vi "Generate Field and Goal Posts.vi"(6 "Height":i16, 11 "Game Board in":refnum<class "Game Board.lvclass">) -> (2 "Goal post out":T1(array[cluster]), 3 "Field limit out":T1(array[cluster]))   [LabVIEW 2021, in "Game Board.lvclass"]
doc: "MIT Licence\nCopyright (c) 2024 David Grollier"
uses:
  Game Board.lvclass
  Game Board.lvclass/Game Board.ctl
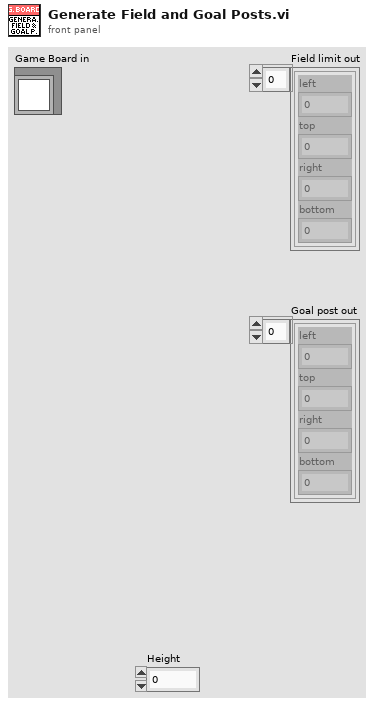
[diagram p1: front panel]
types:
  T1 = cluster{"left":i16, "top":i16, "right":i16, "bottom":i16}[]
  T2 = cluster{"left":i16, "top":i16, "right":i16, "bottom":i16}
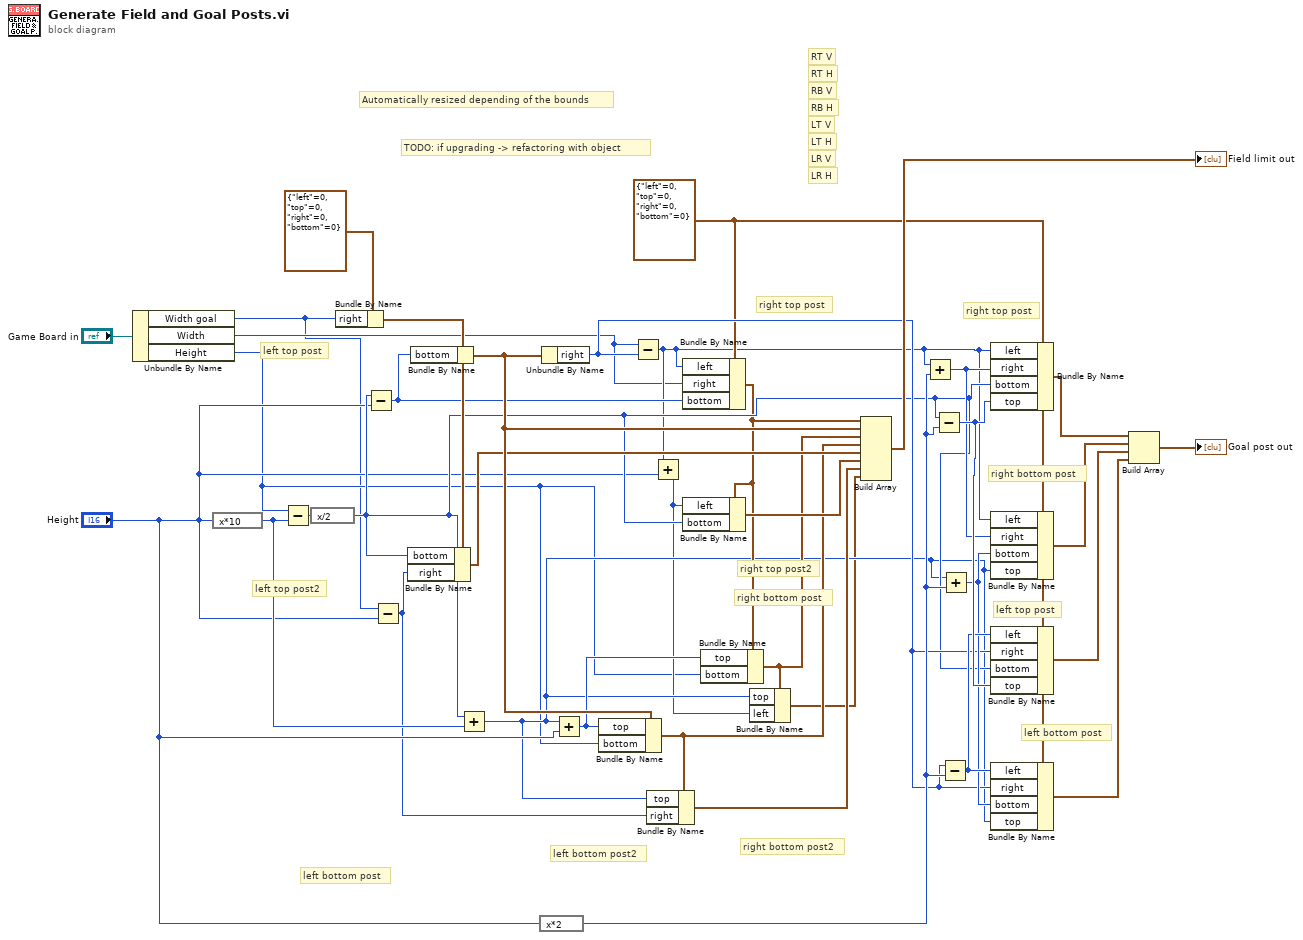
[diagram p0: block diagram]
diagram:
  w18 = T2 {"left"=0, "top"=0, "right"=0, "bottom"=0} ("rect")
  # "TODO: if upgrading -> refactoring with object"
  # "Automatically resized depending of the bounds"
  # "LR H"
  # "LR V"
  # "LT H"
  # "LT V"
  # "RB H"
  # "RB V"
  # "RT H"
  # "RT V"
  # "right bottom post2"
  # "left bottom post2"
  # "right top post2"
  # "left top post2"
  # "left bottom post"
  # "left top post"
  # "right bottom post"
  # "right top post"
  # "left bottom post"
  # "right bottom post"
  # "right top post"
  # "left top post"
  n1 = Unbundle By Name("Game Board in") -> ("Width goal"=w1:u16, "Width"=w3:u32, "Height"=w2:u32)
  n2 = expression code="x*10"("Height") -> (w24:i16)
  n3 = Subtract(x=w2, y=w24) -> (x-y=w23:u32)
  n4 = expression code="x/2"(w23) -> (w17:u32)
  n5 = Bundle By Name(cluster=T2 {"left"=0, "top"=0, "right"=0, "bottom"=0} ("rect"), "right"=w1) -> (w21:T2)
  n6 = Subtract(x=w17, y="Height") -> (x-y=w19:u32)
  n7 = Subtract(x=w1, y="Height") -> (x-y=w11:u16)
  n8 = Bundle By Name(cluster=w21, "bottom"=w17, "right"=w11) -> (w20:T2)
  n9 = Bundle By Name(cluster=w21, "bottom"=w19) -> (w25:T2)
  n10 = Add(x=w17, y=w24) -> (x+y=w7:u32)
  n11 = expression code="x*2"("Height") -> (w27:i16)
  n12 = Unbundle By Name(w25) -> ("right"=w26:i16)
  n13 = Add(x=w7, y="Height") -> (x+y=w9:u32)
  n14 = Bundle By Name(cluster=w25, "top"=w9, "bottom"=w2) -> (w13:T2)
  n15 = Subtract(x=w3, y=w26) -> (x-y=w16:u32)
  n16 = Bundle By Name(cluster=w13, "top"=w7, "right"=w11) -> (w10:T2)
  n17 = Add(x=w16, y="Height") -> (x+y=w6:u32)
  n18 = Bundle By Name(cluster=w18, "left"=w16, "right"=w3, "bottom"=w19) -> (w14:T2)
  n19 = Bundle By Name(cluster=w14, "left"=w6, "bottom"=w17) -> (w15:T2)
  n20 = Bundle By Name(cluster=w14, "top"=w9, "bottom"=w2) -> (w8:T2)
  n21 = Bundle By Name(cluster=w8, "top"=w7, "left"=w6) -> (w5:T2)
  n22 = Build Array(w14, w25, w8, w13, w20, w15, w10, w5) -> (→"Field limit out":T1)
  n23 = Add(x=w16, y=w27) -> (x+y=w29:u32)
  n24 = Subtract(x=w17, y=w27) -> (x-y=w32:u32)
  n25 = Subtract(x=w26, y=w27) -> (x-y=w31:i16)
  n26 = Add(x=w7, y=w27) -> (x+y=w30:u32)
  n27 = Bundle By Name(cluster=w18, "left"=w16, "right"=w29, "bottom"=w17, "top"=w32) -> (w33:T2)
  n28 = Bundle By Name(cluster=w18, "left"=w16, "right"=w29, "bottom"=w30, "top"=w7) -> (w34:T2)
  n29 = Bundle By Name(cluster=w18, "left"=w31, "right"=w26, "bottom"=w17, "top"=w32) -> (w35:T2)
  n30 = Bundle By Name(cluster=w18, "left"=w31, "right"=w26, "bottom"=w30, "top"=w7) -> (w36:T2)
  n31 = Build Array(w33, w34, w35, w36) -> (→"Goal post out":T1)
